vi "_LO_P_OPT2.vi"(5 "_LO_P_OPT":T3={"範囲配列"=[{"Start"=1.0, "Stop"=4.0, "Step"=0.05, "ｂｙ"="NEL VG"}, {"Start"=0.0, "Stop"=100.0, "Step"=4.0, "ｂｙ"="Motor"}, {"Start"=0.0, "Stop"=2.5, "Step"=0.1, "ｂｙ"="WCA VD"}], "Optimize"=0, "file_name"="LP_914.0_Tmin_100519.csv", "Save?"=FALSE, "measure"=1, "current(uA)"=60.0, "wait(ms)"=0, "IFfrq(GHz)"=8.0, "aveg"=10, "SISparam option"=2} {"SISparam option" items=["Volt and Current", "Volt only"]; "measure" items=["Pmax (only HOT)", "Tmin (HOT/COLD)", "C current"]; "Optimize" items=["Sweep", "黄金分割"]; "範囲配列"."Step" format="%.2f"; "範囲配列"."Stop" format="%.2f"; "範囲配列"."Start" format="%.2f"}, 6 "Control":T2={"GPIB_ATT"="28", "6501Dev#"=1, "GPIB_SP"="18", "GPIB_PM"="13", "GPIB_DSA"="11", "GPIB_DMM (TPD)"="23", "GPIB_MPI"="2", "mortor設定"=[{"Axis"=0, "ID"=0, "HIspeed"=200.0, "LOspeed"=100.0, "ACCEL(ms)"=100.0, "Sratio"=50.0, "フリーラン\n"=TRUE, "文字列"="DSB HOT/COLD"}, {"Axis"=1, "ID"=0, "HIspeed"=4.0, "LOspeed"=4.0, "ACCEL(ms)"=100.0, "Sratio"=50.0, "フリーラン\n"=TRUE, "文字列"="SubMM Att"}], "DATAパス"=path "Z:/band10/Labview_ALMA/MIX95/test", "DBパス "=path "Z:/band10/Labview_ALMA/MIX95/test", "comment"="P1_Tmin", "ColdCarts"="003601", "Th"=295.0, "Tc"=77.0, "Set_SIS_volt"=2.1, "Offset"=0.0, "control"=0, "FreqLO"=800.0, "Set_Mag_Cur"=800.0, "MPI offset(mm)"=22.99, "HOT/COLD"=0} {"HOT/COLD" items=["DSB", "SBR", "GainComp"]; "control" items=["CLOSE LOOP", "OPEN LOOP", "Not Control"]}, 7 "Bias_LO_equip":T1={"Node address"=19, "CAN Interface"="CAN0", "Cartridge band"=10, "Slave Node in"={"Address"=19, "Serial Number"=[16, 71, 55, 76, 1, 8, 0, -15]}, "ObjHandle out"=89653312, "POL"=0, "sb"=1, "GPIB_SM (SIS S,V)"="24", "GPIB_DMM (SIS I)"="22", "GPIB_SM (MAG I) "="25", "GPIB_SG(LO)"="19", "GPIB_PW (PAMP) "="6", "GPIB_TMP1(8ch)"="12", "GPIB_TMP2(2ch)  "="13", "WCA_avg"=10, "Rsen"=10.0, "BiasModule"=1, "LOModule "=1, "WCA_LO_FREQ_SET"={"YTO Low freq. [GHz]"=14.42, "YTO High freq. [GHz]"=17.7, "Kvco"=1, "Lock Pol."=0, "SET LO FREQ"=100.0, "Multiplier"=6.0, "YTO (HEX)"=2805, "YTO coarse( FREQ)"=16.666666, "NULL PLL INTEGRATOR"=TRUE}, "Res for"=0} {"Res for" items=["none", "series res", "parallel res"]; "WCA_LO_FREQ_SET"."YTO coarse( FREQ)" min=25 max=150 step=0.0001 format="%.3f"; "WCA_LO_FREQ_SET"."Multiplier" min=3 max=6 step=3; "WCA_LO_FREQ_SET"."SET LO FREQ" min=25 max=150 step=0.0001 format="%.3f"; "WCA_LO_FREQ_SET"."Lock Pol." items=["Lower", "Upper"]; "WCA_LO_FREQ_SET"."Kvco" items=["7.5MHz/V", "15MHz/V"]; "WCA_LO_FREQ_SET"."YTO High freq. [GHz]" format="%.3f"; "WCA_LO_FREQ_SET"."YTO Low freq. [GHz]" format="%.3f"; "LOModule" items=["Manual", "B10Lab LO", "WCA LO"]; "BiasModule" items=["B10Lab Bias", "WCA BiasModule"]; "Slave Node in"."Serial Number" format="%.0x"; "Slave Node in"."Address" format="%.0x"; "Cartridge band" max=10 step=1; "Node address" format="%.0x"}) -> (3 "結果":string="Tmin:1.200000,0.165295,-13.146817,-14.992015,334.790506")   [LabVIEW 2017]
uses:
  __sub_vi/WCA_NAOJ_sub_vi/WCA_Global.vi
panel:
  in  "タブ制御器":enum32{"ページ 1", "ページ 2"}(tab)=enum."ページ 2"
  out "minFx":dbl
  out "Fx":dbl
  out "I-Fx,Pc,Trx":cluster{dbl[], dbl[]}[](graph)=[{[153.7109375, 152.8717041015625, 153.0426025390625, 152.0904541015625, 152.197265625, 151.9866943359375, 151.7333984375, 151.7486572265625, 151.8402099609375, 150.8392333984375, 150.1068115234375, 149.4537353515625, 149.20654296875, 148.6541748046875, 148.1048583984375, 147.0977783203125, 146.6278076171875, 145.062255859375, 144.1864013671875, 143.5546875, 142.291259765625, 140.435791015625, 139.3341064453125, 137.652587890625, 135.430908203125, 133.2977294921875, 131.2896728515625, 129.229736328125, 125.5859375, 122.8668212890625, 118.975830078125, 114.666748046875, 110.8306884765625, 105.0506591796875, 100.1861572265625, 94.15283203125, 88.57421875, 81.0516357421875, 74.462890625, 66.8121337890625, 58.21533203125, 50.9368896484375, 43.5333251953125, 35.0921630859375, 28.1494140625, 21.0784912109375, 16.8365478515625, 13.39111328125, 10.7818603515625, 9.75341796875, 8.4869384765625, 8.978271484375, 8.062744140625, 7.7392578125, 8.43505859375, 7.8125, 7.6416015625, 7.7911376953125, 7.4615478515625, 8.099365234375, 7.89794921875], [247.32973404062736, 244.71794894153766, 242.21978128892934, 244.26842176336262, 241.49817645467988, 244.69487843477683, 242.06455494053583, 240.909445631355, 242.79140491659956, 239.77028849664566, 241.64156684519503, 239.88306106329682, 237.99335929764584, 239.24144610629918, 236.10546909689103, 231.85120086491656, 233.37184450401236, 233.2188877479738, 227.20848640844875, 225.76191805290316, 224.66247085466176, 223.0476471884519, 217.34620955182348, 215.60624700567845, 213.36678724449226, 210.01567868925287, 205.3448700334079, 204.4787981832116, 197.65786587642887, 194.28724400486016, 190.3621373523391, 185.96437875144585, 178.89458547136363, 178.034248343829, 167.74747224652654, 165.5095915634044, 161.1009828285456, 160.72538624241002, 155.93203338638352, 155.50825118261417, 154.03398781536052, 156.39456182240366, 163.7351172921269, 173.95257326151167, 197.43539223873222, 233.31332449649227, 302.2246629701954, 422.0785764312742, 621.6392407626414, 960.4947947838928, 1388.5150609483871, 2060.6013217578993, 2652.2540265629227, 3593.013865996171, 4493.467285194053, 5219.874679791377, 5585.654505061477, 7119.009590999049, 8443.334685028694, 7506.888534465469, 11478.336528646887]}, {[153.7109375, 152.8717041015625, 153.0426025390625, 152.0904541015625, 152.197265625, 151.9866943359375, 151.7333984375, 151.7486572265625, 151.8402099609375, 150.8392333984375, 150.1068115234375, 149.4537353515625, 149.20654296875, 148.6541748046875, 148.1048583984375, 147.0977783203125, 146.6278076171875, 145.062255859375, 144.1864013671875, 143.5546875, 142.291259765625, 140.435791015625, 139.3341064453125, 137.652587890625, 135.430908203125, 133.2977294921875, 131.2896728515625, 129.229736328125, 125.5859375, 122.8668212890625, 118.975830078125, 114.666748046875, 110.8306884765625, 105.0506591796875, 100.1861572265625, 94.15283203125, 88.57421875, 81.0516357421875, 74.462890625, 66.8121337890625, 58.21533203125, 50.9368896484375, 43.5333251953125, 35.0921630859375, 28.1494140625, 21.0784912109375, 16.8365478515625, 13.39111328125, 10.7818603515625, 9.75341796875, 8.4869384765625, 8.978271484375, 8.062744140625, 7.7392578125, 8.43505859375, 7.8125, 7.6416015625, 7.7911376953125, 7.4615478515625, 8.099365234375, 7.89794921875], [-14.7646696, -14.7654326, -14.7765426, -14.7599957, -14.7587965, -14.7416571, -14.7490545, -14.7393598, -14.7286239, -14.7227317, -14.7104064, -14.7025198, -14.6874695, -14.6799035, -14.6761139, -14.6736071, -14.6591382, -14.6331242, -14.6237809, -14.6066206, -14.5690542, -14.5442752, -14.5291663, -14.508835, -14.4645891, -14.4304201, -14.3839625, -14.3296729, -14.3047591, -14.2758504, -14.2368317, -14.1673127, -14.1313886, -14.0570048, -14.0333737, -13.9726864, -13.9307766, -13.8943843, -13.9278091, -13.9695187, -14.0952793, -14.286396, -14.5693598, -14.9860507, -15.5360188, -16.2362229, -17.0032381, -17.7253118, -18.2916002, -18.6658912, -18.9074033, -19.0515672, -19.1514628, -19.2030341, -19.2343409, -19.256989, -19.2916912, -19.2884725, -19.3062143, -19.3276449, -19.3006641]}, {[153.7109375, 152.8717041015625, 153.0426025390625, 152.0904541015625, 152.197265625, 151.9866943359375, 151.7333984375, 151.7486572265625, 151.8402099609375, 150.8392333984375, 150.1068115234375, 149.4537353515625, 149.20654296875, 148.6541748046875, 148.1048583984375, 147.0977783203125, 146.6278076171875, 145.062255859375, 144.1864013671875, 143.5546875, 142.291259765625, 140.435791015625, 139.3341064453125, 137.652587890625, 135.430908203125, 133.2977294921875, 131.2896728515625, 129.229736328125, 125.5859375, 122.8668212890625, 118.975830078125, 114.666748046875, 110.8306884765625, 105.0506591796875, 100.1861572265625, 94.15283203125, 88.57421875, 81.0516357421875, 74.462890625, 66.8121337890625, 58.21533203125, 50.9368896484375, 43.5333251953125, 35.0921630859375, 28.1494140625, 21.0784912109375, 16.8365478515625, 13.39111328125, 10.7818603515625, 9.75341796875, 8.4869384765625, 8.978271484375, 8.062744140625, 7.7392578125, 8.43505859375, 7.8125, 7.6416015625, 7.7911376953125, 7.4615478515625, 8.099365234375, 7.89794921875], [247.32973404062736, 244.71794894153766, 242.21978128892934, 244.26842176336262, 241.49817645467988, 244.69487843477683, 242.06455494053583, 240.909445631355, 242.79140491659956, 239.77028849664566, 241.64156684519503, 239.88306106329682, 237.99335929764584, 239.24144610629918, 236.10546909689103, 231.85120086491656, 233.37184450401236, 233.2188877479738, 227.20848640844875, 225.76191805290316, 224.66247085466176, 223.0476471884519, 217.34620955182348, 215.60624700567845, 213.36678724449226, 210.01567868925287, 205.3448700334079, 204.4787981832116, 197.65786587642887, 194.28724400486016, 190.3621373523391, 185.96437875144585, 178.89458547136363, 178.034248343829, 167.74747224652654, 165.5095915634044, 161.1009828285456, 160.72538624241002, 155.93203338638352, 155.50825118261417, 154.03398781536052, 156.39456182240366, 163.7351172921269, 173.95257326151167, 197.43539223873222, 233.31332449649227, 302.2246629701954, 422.0785764312742, 621.6392407626414, 960.4947947838928, 1388.5150609483871, 2060.6013217578993, 2652.2540265629227, 3593.013865996171, 4493.467285194053, 5219.874679791377, 5585.654505061477, 7119.009590999049, 8443.334685028694, 7506.888534465469, 11478.336528646887]}]
  out "X-I,Fx":cluster{dbl[], dbl[]}[](graph)=[{[1.0, 1.05, 1.1, 1.15, 1.2, 1.25, 1.3, 1.35, 1.4, 1.45, 1.5, 1.55, 1.6, 1.65, 1.7000000000000002, 1.75, 1.8, 1.85, 1.9, 1.9500000000000002, 2.0, 2.05, 2.1, 2.1500000000000004, 2.2, 2.25, 2.3, 2.35, 2.4000000000000004, 2.45, 2.5, 2.55, 2.6, 2.6500000000000004, 2.7, 2.75, 2.8, 2.85, 2.9000000000000004, 2.95, 3.0, 3.0500000000000003, 3.1, 3.15, 3.2, 3.25, 3.3000000000000003, 3.35, 3.4000000000000004, 3.45, 3.5, 3.5500000000000003, 3.6, 3.6500000000000004, 3.7, 3.75, 3.8000000000000003, 3.85, 3.9000000000000004, 3.95, 4.0], [153.7109375, 152.8717041015625, 153.0426025390625, 152.0904541015625, 152.197265625, 151.9866943359375, 151.7333984375, 151.7486572265625, 151.8402099609375, 150.8392333984375, 150.1068115234375, 149.4537353515625, 149.20654296875, 148.6541748046875, 148.1048583984375, 147.0977783203125, 146.6278076171875, 145.062255859375, 144.1864013671875, 143.5546875, 142.291259765625, 140.435791015625, 139.3341064453125, 137.652587890625, 135.430908203125, 133.2977294921875, 131.2896728515625, 129.229736328125, 125.5859375, 122.8668212890625, 118.975830078125, 114.666748046875, 110.8306884765625, 105.0506591796875, 100.1861572265625, 94.15283203125, 88.57421875, 81.0516357421875, 74.462890625, 66.8121337890625, 58.21533203125, 50.9368896484375, 43.5333251953125, 35.0921630859375, 28.1494140625, 21.0784912109375, 16.8365478515625, 13.39111328125, 10.7818603515625, 9.75341796875, 8.4869384765625, 8.978271484375, 8.062744140625, 7.7392578125, 8.43505859375, 7.8125, 7.6416015625, 7.7911376953125, 7.4615478515625, 8.099365234375, 7.89794921875]}, {[1.0, 1.05, 1.1, 1.15, 1.2, 1.25, 1.3, 1.35, 1.4, 1.45, 1.5, 1.55, 1.6, 1.65, 1.7000000000000002, 1.75, 1.8, 1.85, 1.9, 1.9500000000000002, 2.0, 2.05, 2.1, 2.1500000000000004, 2.2, 2.25, 2.3, 2.35, 2.4000000000000004, 2.45, 2.5, 2.55, 2.6, 2.6500000000000004, 2.7, 2.75, 2.8, 2.85, 2.9000000000000004, 2.95, 3.0, 3.0500000000000003, 3.1, 3.15, 3.2, 3.25, 3.3000000000000003, 3.35, 3.4000000000000004, 3.45, 3.5, 3.5500000000000003, 3.6, 3.6500000000000004, 3.7, 3.75, 3.8000000000000003, 3.85, 3.9000000000000004, 3.95, 4.0], [247.32973404062736, 244.71794894153766, 242.21978128892934, 244.26842176336262, 241.49817645467988, 244.69487843477683, 242.06455494053583, 240.909445631355, 242.79140491659956, 239.77028849664566, 241.64156684519503, 239.88306106329682, 237.99335929764584, 239.24144610629918, 236.10546909689103, 231.85120086491656, 233.37184450401236, 233.2188877479738, 227.20848640844875, 225.76191805290316, 224.66247085466176, 223.0476471884519, 217.34620955182348, 215.60624700567845, 213.36678724449226, 210.01567868925287, 205.3448700334079, 204.4787981832116, 197.65786587642887, 194.28724400486016, 190.3621373523391, 185.96437875144585, 178.89458547136363, 178.034248343829, 167.74747224652654, 165.5095915634044, 161.1009828285456, 160.72538624241002, 155.93203338638352, 155.50825118261417, 154.03398781536052, 156.39456182240366, 163.7351172921269, 173.95257326151167, 197.43539223873222, 233.31332449649227, 302.2246629701954, 422.0785764312742, 621.6392407626414, 960.4947947838928, 1388.5150609483871, 2060.6013217578993, 2652.2540265629227, 3593.013865996171, 4493.467285194053, 5219.874679791377, 5585.654505061477, 7119.009590999049, 8443.334685028694, 7506.888534465469, 11478.336528646887]}]
  out "Link済み":bool
  # "LO freq. [GHz]"
  # "YTO LOW\n/High Freq."
  # "ZERO Intgrtr"
  # "Node Address"
  # "Serial Number"
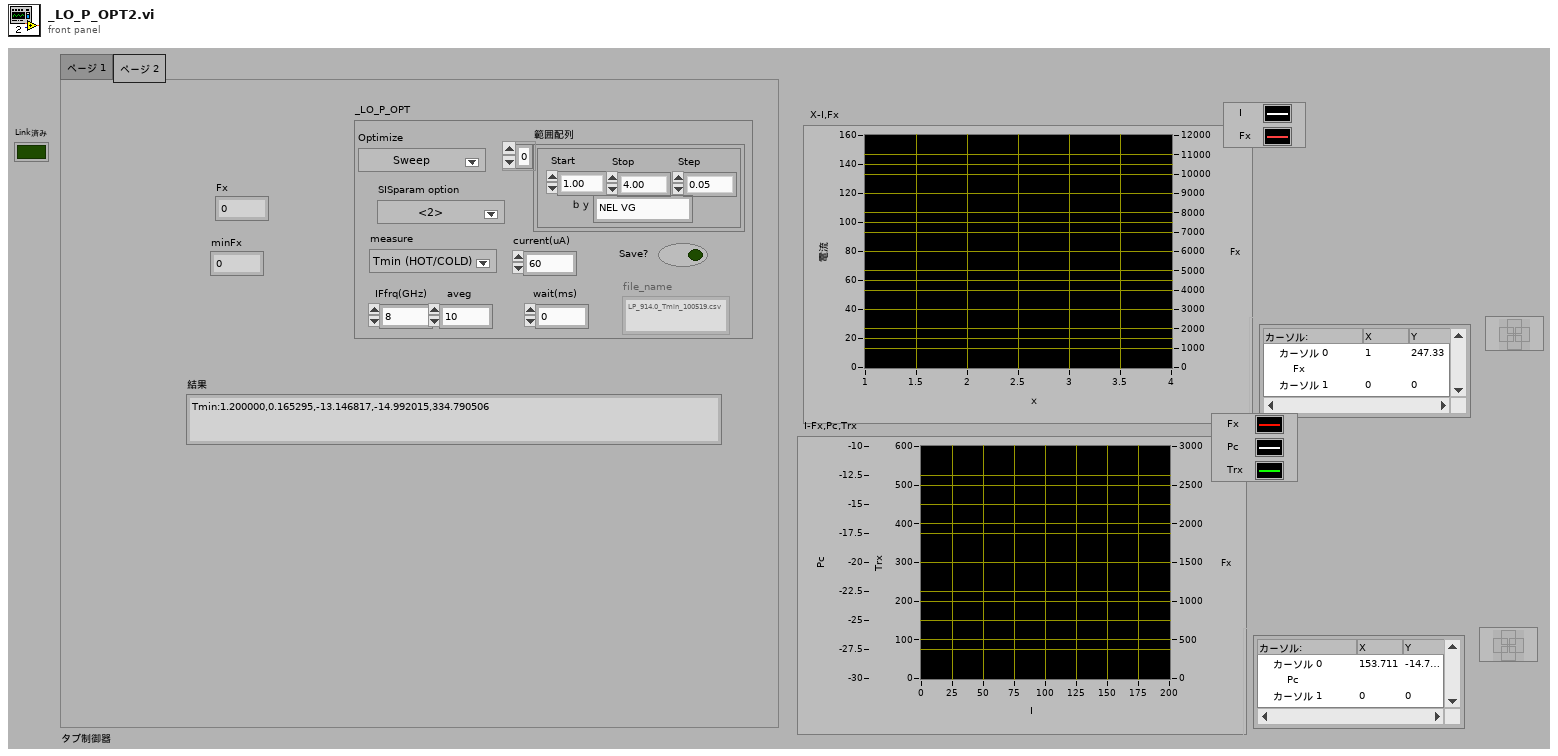
[diagram p1: front panel]
types:
  T1 = cluster{"Node address":u16, "CAN Interface":string, "Cartridge band":u32, "Slave Node in":cluster{"Address":i16, "Serial Number":i8[]}, "ObjHandle out":u32, "POL":u32, "sb":u32, "GPIB_SM (SIS S,V)":string, "GPIB_DMM (SIS I)":string, "GPIB_SM (MAG I) ":string, "GPIB_SG(LO)":string, "GPIB_PW (PAMP) ":string, "GPIB_TMP1(8ch)":string, "GPIB_TMP2(2ch)  ":string, "WCA_avg":i32, "Rsen":dbl, "BiasModule":u16, "LOModule ":u16, "WCA_LO_FREQ_SET":cluster{"YTO Low freq. [GHz]":sgl, "YTO High freq. [GHz]":sgl, "Kvco":u16, "Lock Pol.":u16, "SET LO FREQ":sgl, "Multiplier":sgl, "YTO (HEX)":u16, "YTO coarse( FREQ)":sgl, "NULL PLL INTEGRATOR":bool}, "Res for":u16}
  T2 = cluster{"GPIB_ATT":string, "6501Dev#":i16, "GPIB_SP":string, "GPIB_PM":string, "GPIB_DSA":string, "GPIB_DMM (TPD)":string, "GPIB_MPI":string, "mortor設定":cluster{"Axis":i16, "ID":i16, "HIspeed":dbl, "LOspeed":dbl, "ACCEL(ms)":dbl, "Sratio":dbl, "フリーラン\n":bool, "文字列":string}[], "DATAパス":path, "DBパス ":path, "comment":string, "ColdCarts":string, "Th":dbl, "Tc":dbl, "Set_SIS_volt":dbl, "Offset":dbl, "control":u16, "FreqLO":dbl, "Set_Mag_Cur":dbl, "MPI offset(mm)":dbl, "HOT/COLD":u16}
  T3 = cluster{"範囲配列":cluster{"Start":dbl, "Stop":dbl, "Step":dbl, "ｂｙ":string}[], "Optimize":u16, "file_name":string, "Save?":bool, "measure":u16, "current(uA)":dbl, "wait(ms)":i32, "IFfrq(GHz)":dbl, "aveg":i32, "SISparam option":u16}
  T4 = cluster{"Axis":i16, "ID":i16, "HIspeed":dbl, "LOspeed":dbl, "ACCEL(ms)":dbl, "Sratio":dbl, "フリーラン\n":bool, "文字列":string}[]
  T5 = cluster{"Axis":i16, "ID":i16, "HIspeed":dbl, "LOspeed":dbl, "ACCEL(ms)":dbl, "Sratio":dbl, "フリーラン\n":bool, "文字列":string}
  T6 = cluster{"Start":dbl, "Stop":dbl, "Step":dbl, "ｂｙ":string}[]
  T7 = cluster{"Start":dbl, "Stop":dbl, "Step":dbl, "ｂｙ":string}
  T8 = cluster{"PA_A_DRAIN_V":sgl, "PA_A_DRAIN_C":sgl, "PA_A_GATE_V":sgl, "PA_B_DRAIN_V":sgl, "PA_B_DRAIN_C":sgl, "PA_B_GATE_V":sgl, "PA_3V_SUPPLY_V":sgl, "PA_5V_MON":sgl}
  T9 = cluster{"出力配列[0]":dbl, "出力配列[1]":dbl, "出力配列[2]":dbl, "出力配列[3]":dbl, "出力配列[4]":dbl, "出力配列[5]":dbl, "出力配列[6]":dbl}
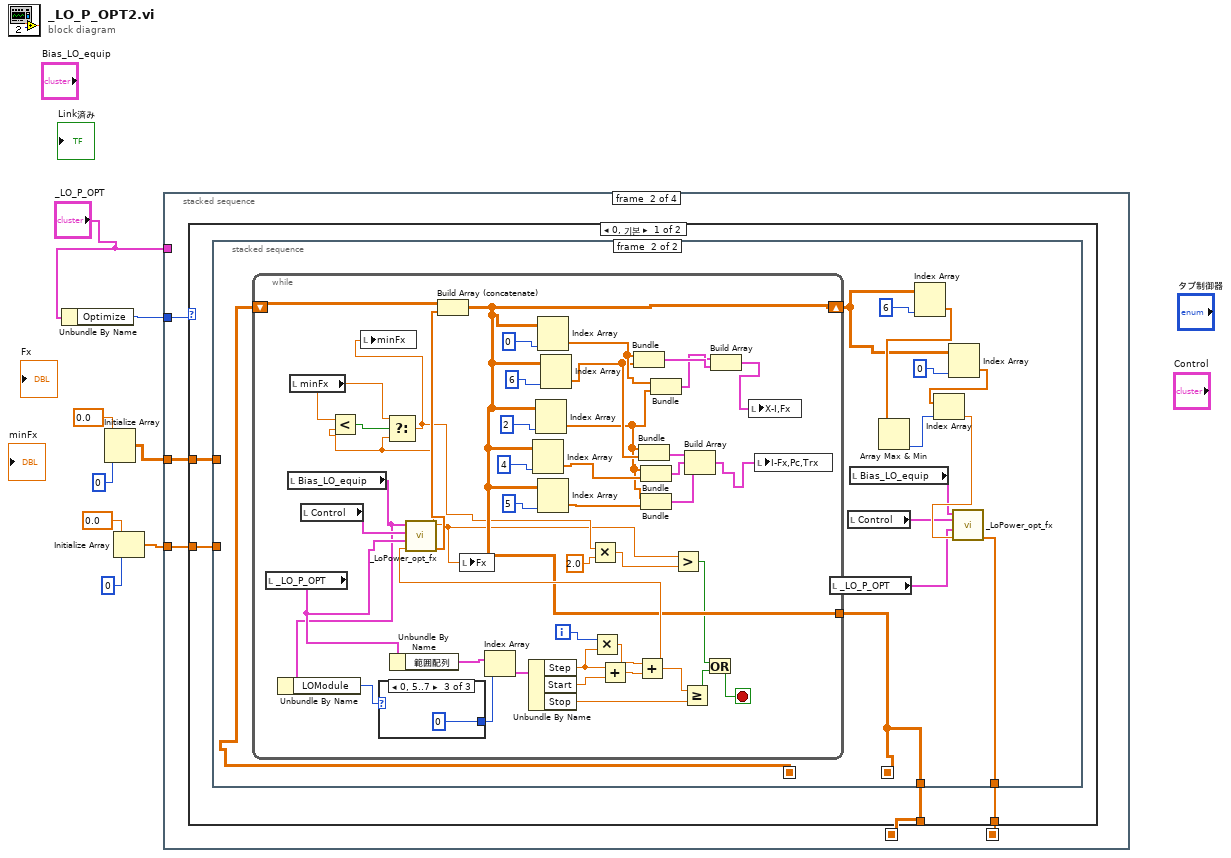
[diagram p0: block diagram]
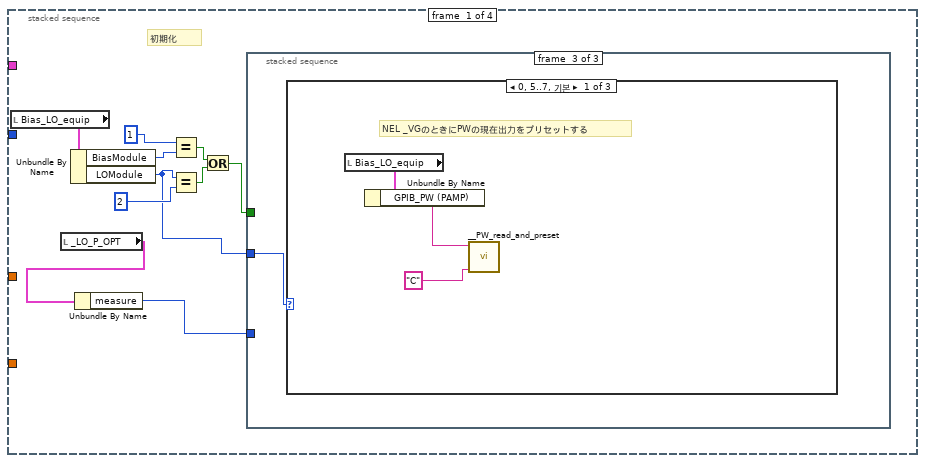
[diagram p2: hidden frame]
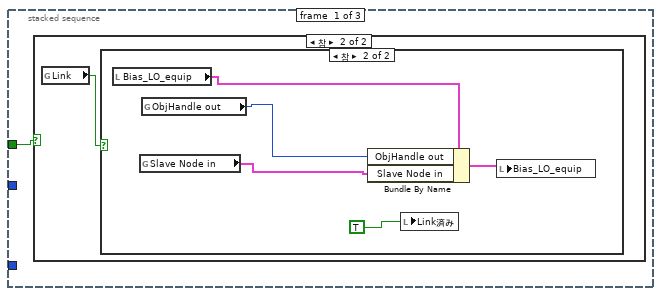
[diagram p3: hidden frame]
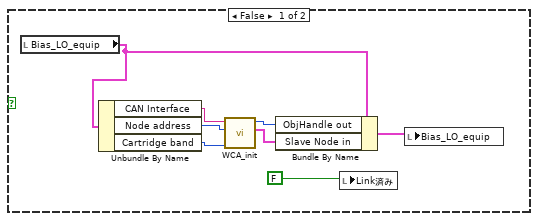
[diagram p5: hidden frame]
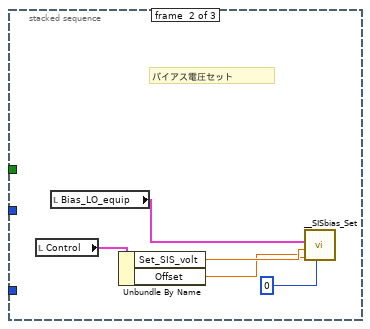
[diagram p6: hidden frame]
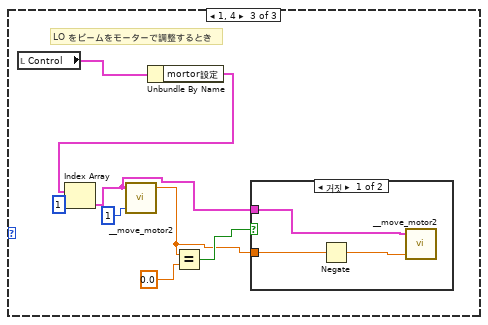
[diagram p8: hidden frame]
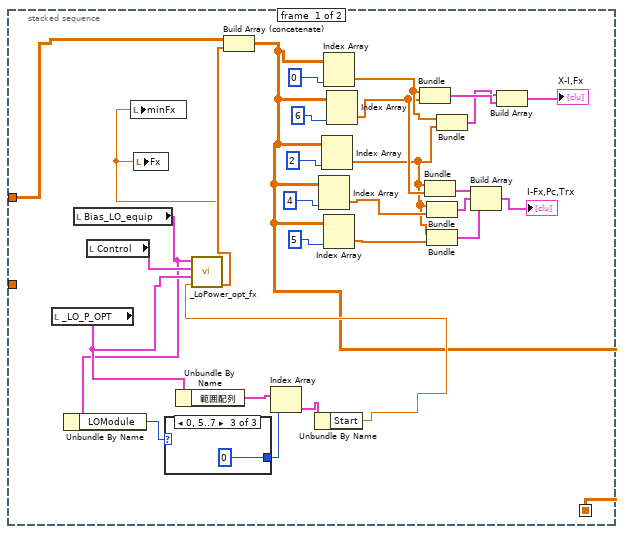
[diagram p10: hidden frame]
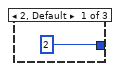
[diagram p11: hidden frame]
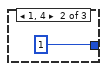
[diagram p12: hidden frame]
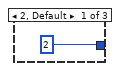
[diagram p13: hidden frame]
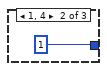
[diagram p14: hidden frame]
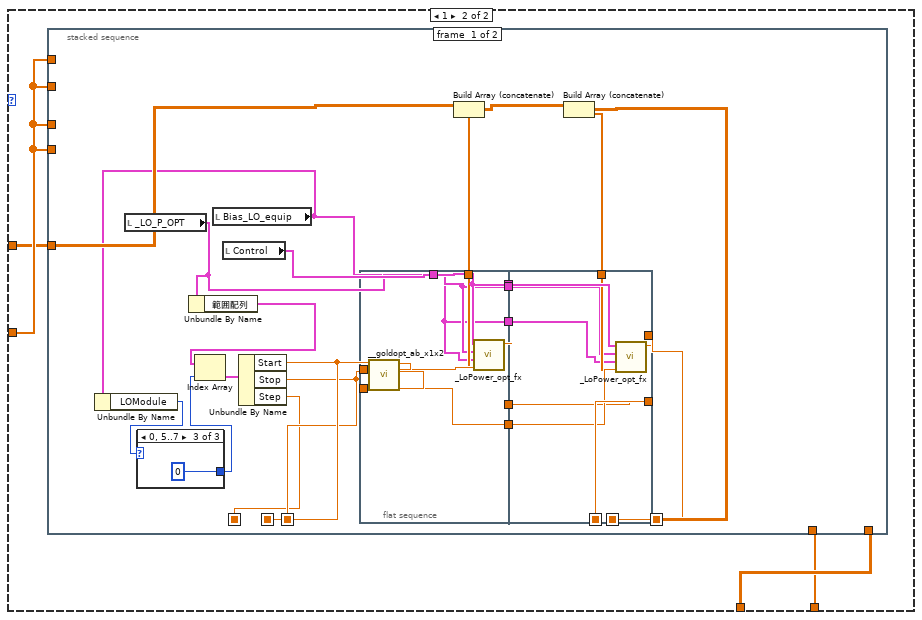
[diagram p15: hidden frame]
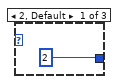
[diagram p16: hidden frame]
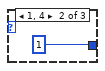
[diagram p17: hidden frame]
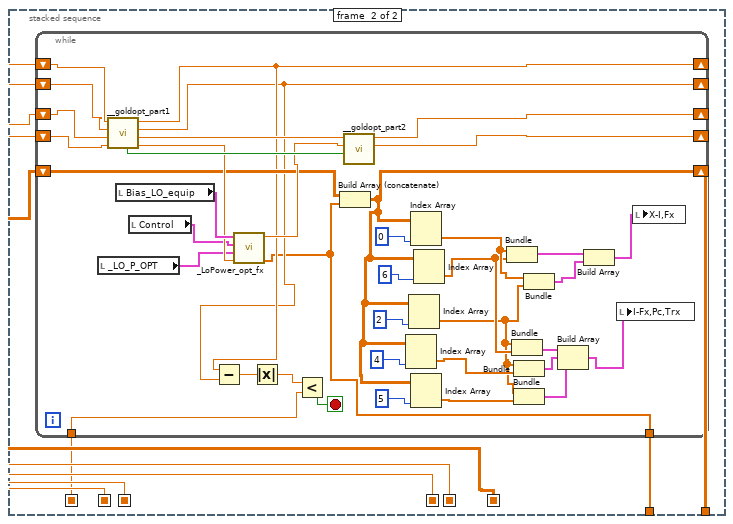
[diagram p18: hidden frame]
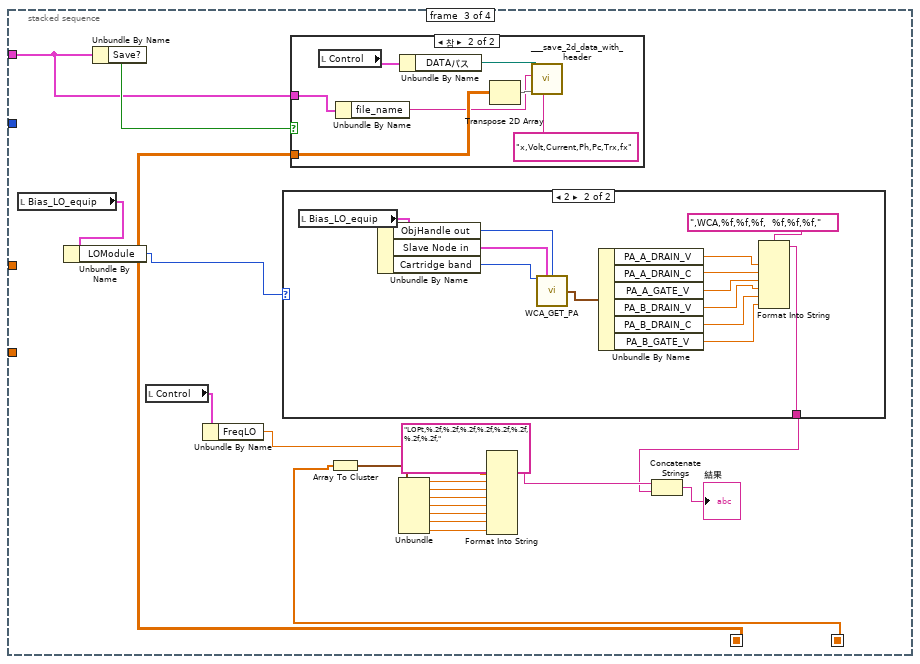
[diagram p19: hidden frame]
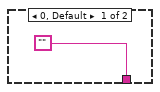
[diagram p20: hidden frame]
diagram:
  w2 = 0
  n1 = Unbundle By Name("_LO_P_OPT") -> ("Optimize"=w4:u16)
  n2 = Initialize Array(0.0, w2, w2) -> (w1:dbl[][])
  n3 = Initialize Array(0.0, 0) -> (w6:dbl[])
  n4 = stacked-sequence {
    seq-local: [_ w56 _ _] -> [_ _ w264 _]
    seq-local: [_ w54 _ _] -> [_ _ w262 _]
    tunnel: w6 -> [_ w57 _ _]
    tunnel: "_LO_P_OPT" -> [_ _ w263 _]
    tunnel: w4 -> [_ w58 _ _]
    tunnel: w1 -> [_ w55 _ _]
    frame #0 {
      # "初期化"
      n5 = local read "Bias_LO_equip"() -> (w13:T1)
      n6 = local read "_LO_P_OPT"() -> (w11:T3)
      n7 = Unbundle By Name(w13) -> ("BiasModule"=w14:u16, "LOModule"=w9:u16)
      n8 = Unbundle By Name(w11) -> ("measure"=w10:u16)
      n9 = Equal?(x=1, y=w14) -> (x = y?=w17:bool)
      n10 = Equal?(x=w9, y=2) -> (x = y?=w18:bool)
      n11 = Or(x=w17, y=w18) -> (x .or. y?=w12:bool)
      n12 = stacked-sequence {
        tunnel: w12 -> [w19 _ _]
        tunnel: w10 -> [_ _ _]
        tunnel: w9 -> [_ _ w39]
        frame #0 {
          n13 = case shown="참" w19 {
            frame False {
            }
            frame True {
              n14 = global read "WCA_Global.vi" "Link"() -> (w20:bool)
              n15 = case shown="참" w20 {
                frame False {
                  n16 = local read "Bias_LO_equip"() -> (w22:T1)
                  n17 = Unbundle By Name(w22) -> ("CAN Interface"=w26:string, "Node address"=w25:u16, "Cartridge band"=w24:u32)
                  n18 = call "WCA_init.vi"("Cartridge band"=w24, "Node address"=w25, "CAN Interface"=w26) -> ("Slave Node in"=w27:cluster{"Address":i16, "Serial Number":i8[]}, "ObjHandle out"=w28:u32)  [unwired: 4 in, 3 out]
                  n19 = Bundle By Name(cluster=w22, "ObjHandle out"=w28, "Slave Node in"=w27) -> (w23:T1)
                  n20 = local write "Link済み"(FALSE) -> ()
                  n21 = local write "Bias_LO_equip"(w23) -> ()
                }
                frame True {
                  n22 = local read "Bias_LO_equip"() -> (w32:T1)
                  n23 = global read "WCA_Global.vi" "Slave Node in"() -> (w30:cluster{"Address":i16, "Serial Number":i8[]})
                  n24 = global read "WCA_Global.vi" "ObjHandle out"() -> (w31:u32)
                  n25 = Bundle By Name(cluster=w32, "ObjHandle out"=w31, "Slave Node in"=w30) -> (w33:T1)
                  n26 = local write "Link済み"(TRUE) -> ()
                  n27 = local write "Bias_LO_equip"(w33) -> ()
                }
              }
            }
          }
        }
        frame #1 {
          # "バイアス電圧セット"
          n28 = local read "Control"() -> (w36:T2)
          n29 = local read "Bias_LO_equip"() -> (w38:T1)
          n30 = Unbundle By Name(w36) -> ("Set_SIS_volt"=w35:dbl, "Offset"=w34:dbl)
          n31 = call "__SISbias_Set.vi"("SIS　Mode"=0, "Offset"=w34, "Set_V"=w35, "Bias_LO_equip"=w38) -> ()  [unwired: 7 in, 1 out]
        }
        frame #2 {
          n32 = case shown="0, 5..7, 기본" w39 {
            frame 0, 5..7, Default {
              # "NEL _VGのときにPWの現在出力をプリセットする"
              n33 = local read "Bias_LO_equip"() -> (w42:T1)
              n34 = Unbundle By Name(w42) -> ("GPIB_PW (PAMP)"=w41:string)
              n35 = call "__PW_read_and_preset.vi"("MAXCh（A,B,C,D）"="C", "GPIB"=w41) -> ()  [unwired: 10 in]
            }
            frame 2 {
            }
            frame 1, 4 {
              # "LO をビームをモーターで調整するとき"
              n36 = local read "Control"() -> (w47:T2)
              n37 = Unbundle By Name(w47) -> ("mortor設定"=w48:T4)
              n38 = Index Array(array=w48, index=1) -> (element=w43:T5)
              n39 = call "__move_motor2.vi"("Moving distance"=1, "motor setup"=w43) -> ("counter"=w44:dbl)  [unwired: 2 in, 1 out]
              n40 = Equal?(x=w44, y=0.0) -> (x = y?=w50:bool)
              n41 = case shown="거짓" w50 {
                tunnel: w44 -> [w53 _]
                tunnel: w43 -> [w51 _]
                frame False {
                  n42 = Negate(x=w53) -> (-x=w52:dbl)
                  n43 = call "__move_motor2.vi"("Moving distance"=w52, "motor setup"=w51) -> ()  [unwired: 2 in, 2 out]
                }
                frame True {
                }
              }
            }
          }
        }
      }
    }
    frame #1 {
      n44 = case shown="0, 기본" w58 {
        tunnel: w57 -> [w62 w157]
        tunnel: [w61 w155] -> w56
        tunnel: w55 -> [w60 w156]
        tunnel: [w59 w154] -> w54
        frame 0, Default {
          n45 = stacked-sequence {
            seq-local: [_ w105] -> [_ _]
            seq-local: [w64 _] -> [_ w95]
            tunnel: w62 -> [_ _]
            tunnel: [_ w105] -> w61
            tunnel: w60 -> [w91 _]
            tunnel: [_ w97] -> w59
            frame #0 {
              n46 = local read "_LO_P_OPT"() -> (w69:T3)
              n47 = local read "Bias_LO_equip"() -> (w68:T1)
              n48 = Unbundle By Name(w68) -> ("LOModule"=w67:u16)
              n49 = local read "Control"() -> (w70:T2)
              n50 = case shown="0, 5..7" w67 {
                tunnel: [2 1 0] -> w66
                frame 2, Default {
                }
                frame 1, 4 {
                }
                frame 0, 5..7 {
                }
              }
              n51 = Unbundle By Name(w69) -> ("範囲配列"=w90:T6)
              n52 = Index Array(array=w90, index=w66) -> (element=w89:T7)
              n53 = Unbundle By Name(w89) -> ("Start"=w65:dbl)
              n54 = call "_LoPower_opt_fx.vi"("ｘ"=w65, "_LO_P_OPT"=w69, "Control"=w70, "Bias_LO_equip"=w68) -> ("出力配列"=w85:dbl[], "fx"=w63:dbl)  [unwired: 6 in]
              n55 = local write "minFx"(w63) -> ()
              n56 = local write "Fx"(w63) -> ()
              n57 = Build Array (concatenate)(w91, w85) -> (w64:dbl[][])
              n58 = Index Array(array=w64, index (col)=4) -> (element=w81:dbl[])  [unwired: 1 in]
              n59 = Index Array(array=w64, index (col)=2) -> (element=w80:dbl[])  [unwired: 1 in]
              n60 = Index Array(array=w64, index (col)=0) -> (element=w84:dbl[])  [unwired: 1 in]
              n61 = Index Array(array=w64, index (col)=5) -> (element=w79:dbl[])  [unwired: 1 in]
              n62 = Index Array(array=w64, index (col)=6) -> (element=w82:dbl[])  [unwired: 1 in]
              n63 = Bundle(w84, w82) -> (w72:cluster{dbl[], dbl[]})  [unwired: 1 in]
              n64 = Bundle(w80, w82) -> (w88:cluster{dbl[], dbl[]})  [unwired: 1 in]
              n65 = Bundle(w80, w81) -> (w87:cluster{dbl[], dbl[]})  [unwired: 1 in]
              n66 = Bundle(w80, w79) -> (w86:cluster{dbl[], dbl[]})  [unwired: 1 in]
              n67 = Bundle(w84, w80) -> (w71:cluster{dbl[], dbl[]})  [unwired: 1 in]
              n68 = Build Array(w88, w87, w86) -> (→"I-Fx,Pc,Trx":cluster{dbl[], dbl[]}[])
              n69 = Build Array(w71, w72) -> (→"X-I,Fx":cluster{dbl[], dbl[]}[])
            }
            frame #1 {
              n70 = while {
                tunnel: [w138] -> w105
                shift-right: [w138] -> w99
                shift-left: w95 -> [w140]
                i -> [w147]
                stop <- w115 stop-if-true
                n71 = local read "_LO_P_OPT"() -> (w124:T3)
                n72 = local read "Bias_LO_equip"() -> (w123:T1)
                n73 = Unbundle By Name(w123) -> ("LOModule"=w122:u16)
                n74 = local read "minFx"() -> (w117:dbl)
                n75 = local read "Control"() -> (w125:T2)
                n76 = case shown="0, 5..7" w122 {
                  tunnel: [2 1 0] -> w121
                  frame 2, Default {
                  }
                  frame 1, 4 {
                  }
                  frame 0, 5..7 {
                  }
                }
                n77 = Unbundle By Name(w124) -> ("範囲配列"=w150:T6)
                n78 = Index Array(array=w150, index=w121) -> (element=w149:T7)
                n79 = Unbundle By Name(w149) -> ("Step"=w119:dbl, "Start"=w148:dbl, "Stop"=w145:dbl)
                n80 = Multiply(x=w147, y=w119) -> (x*y=w146:dbl)
                n81 = Add(x=w119, y=w148) -> (x+y=w120:dbl)
                n82 = Add(x=w146, y=w120) -> (x+y=w144:dbl)
                n83 = call "_LoPower_opt_fx.vi"("ｘ"=w144, "_LO_P_OPT"=w124, "Control"=w125, "Bias_LO_equip"=w123) -> ("出力配列"=w139:dbl[], "fx"=w111:dbl)  [unwired: 6 in]
                n84 = Less?(x=w117, y=w111) -> (x < y?=w118:bool)
                n85 = Select(t=w117, s=w118, f=w111) -> (s? t:f=w112:dbl)
                n86 = local write "minFx"(w112) -> ()
                n87 = Build Array (concatenate)(w140, w139) -> (w138:dbl[][])
                n88 = local write "Fx"(w111) -> ()
                n89 = Index Array(array=w138, index (col)=4) -> (element=w135:dbl[])  [unwired: 1 in]
                n90 = Index Array(array=w138, index (col)=2) -> (element=w134:dbl[])  [unwired: 1 in]
                n91 = Index Array(array=w138, index (col)=0) -> (element=w137:dbl[])  [unwired: 1 in]
                n92 = Index Array(array=w138, index (col)=5) -> (element=w133:dbl[])  [unwired: 1 in]
                n93 = Index Array(array=w138, index (col)=6) -> (element=w136:dbl[])  [unwired: 1 in]
                n94 = Multiply(x=w112, y=2.0) -> (x*y=w110:dbl)
                n95 = Bundle(w137, w136) -> (w127:cluster{dbl[], dbl[]})  [unwired: 1 in]
                n96 = Bundle(w134, w136) -> (w143:cluster{dbl[], dbl[]})  [unwired: 1 in]
                n97 = Bundle(w134, w135) -> (w142:cluster{dbl[], dbl[]})  [unwired: 1 in]
                n98 = Bundle(w134, w133) -> (w141:cluster{dbl[], dbl[]})  [unwired: 1 in]
                n99 = Bundle(w137, w134) -> (w126:cluster{dbl[], dbl[]})  [unwired: 1 in]
                n100 = Greater?(x=w111, y=w110) -> (0:w113:bool)
                n101 = Greater Or Equal?(x=w144, y=w145) -> (x >= y?=w114:bool)
                n102 = Build Array(w143, w142, w141) -> (w108:cluster{dbl[], dbl[]}[])
                n103 = Or(x=w113, y=w114) -> (x .or. y?=w115:bool)
                n104 = Build Array(w126, w127) -> (w109:cluster{dbl[], dbl[]}[])
                n105 = local write "X-I,Fx"(w109) -> ()
                n106 = local write "I-Fx,Pc,Trx"(w108) -> ()
              }
              n107 = local read "_LO_P_OPT"() -> (w96:T3)
              n108 = local read "Control"() -> (w100:T2)
              n109 = local read "Bias_LO_equip"() -> (w106:T1)
              n110 = Index Array(array=w99, index (col)=6) -> (element=w104:dbl[])  [unwired: 1 in]
              n111 = Array Max & Min(array=w104) -> (min index (indices)=w98:i32)  [unwired: 3 out]
              n112 = Index Array(array=w99, index (col)=0) -> (element=w103:dbl[])  [unwired: 1 in]
              n113 = Index Array(array=w103, index=w98) -> (element=w107:dbl)
              n114 = call "_LoPower_opt_fx.vi"("ｘ"=w107, "_LO_P_OPT"=w96, "Control"=w100, "Bias_LO_equip"=w106) -> ("出力配列"=w97:dbl[])  [unwired: 6 in, 1 out]
            }
          }
        }
        frame 1 {
          n115 = stacked-sequence {
            seq-local: [w169 _] -> [_ w206]
            seq-local: [w168 _] -> [_ w205]
            seq-local: [w171 _] -> [_ w202]
            seq-local: [w166 _] -> [_ w204]
            seq-local: [w165 _] -> [_ w203]
            seq-local: [w164 _] -> [_ w201]
            tunnel: w157 -> [_ _]
            tunnel: w157 -> [_ _]
            tunnel: w157 -> [_ _]
            tunnel: w157 -> [_ _]
            tunnel: w156 -> [w176 _]
            tunnel: [_ w200] -> w155
            tunnel: [_ w199] -> w154
            frame #0 {
              n116 = local read "_LO_P_OPT"() -> (w162:T3)
              n117 = Unbundle By Name(w162) -> ("範囲配列"=w181:T6)
              n118 = local read "Bias_LO_equip"() -> (w158:T1)
              n119 = Unbundle By Name(w158) -> ("LOModule"=w159:u16)
              n120 = case shown="0, 5..7" w159 {
                tunnel: [2 1 0] -> w160
                frame 2, Default {
                }
                frame 1, 4 {
                }
                frame 0, 5..7 {
                }
              }
              n121 = Index Array(array=w181, index=w160) -> (element=w180:T7)
              n122 = local read "Control"() -> (w179:T2)
              n123 = Unbundle By Name(w180) -> ("Start"=w169:dbl, "Stop"=w168:dbl, "Step"=w164:dbl)
              n124 = flat-sequence {
                tunnel: w162 -> [w185]
                tunnel: w179 -> [w186]
                tunnel: w158 -> [w190]
                tunnel: w172 -> [w191]
                tunnel: [w190] -> w178
                tunnel: w170 -> [w189]
                tunnel: [w189] -> w177
                tunnel: [w188] -> w175
                tunnel: [w187] -> w167
                tunnel: [w186] -> w163
                tunnel: [w185] -> w161
                tunnel: w178 -> [w198]
                tunnel: w177 -> [w197]
                tunnel: [w196] -> w173
                tunnel: w167 -> [w195]
                tunnel: [w195] -> w166
                tunnel: [w194] -> w165
                tunnel: w163 -> [w193]
                tunnel: w161 -> [w192]
                frame #0 {
                  n125 = call "_LoPower_opt_fx.vi"("ｘ"=w191, "_LO_P_OPT"=w185, "Control"=w186, "Bias_LO_equip"=w190) -> ("出力配列"=w188:dbl[], "fx"=w187:dbl)  [unwired: 6 in]
                }
                frame #1 {
                  n126 = call "_LoPower_opt_fx.vi"("ｘ"=w197, "_LO_P_OPT"=w192, "Control"=w193, "Bias_LO_equip"=w198) -> ("出力配列"=w196:dbl[], "fx"=w194:dbl)  [unwired: 6 in]
                }
              }
              n127 = call "__goldopt_ab_x1x2.vi"("bi"=w168, "ai"=w169) -> ("x2"=w170:dbl, "x1"=w172:dbl)  [unwired: 8 in]
              n128 = Build Array (concatenate)(w176, w175) -> (w174:dbl[][])
              n129 = Build Array (concatenate)(w174, w173) -> (w171:dbl[][])
            }
            frame #1 {
              n130 = while {
                shift-right: [w214] -> _
                shift-left: w206 -> [w245]
                shift-right: [w213] -> _
                shift-left: w205 -> [w244]
                shift-right: [w236] -> _
                shift-left: w204 -> [w243]
                shift-right: [w235] -> _
                shift-left: w203 -> [w242]
                shift-right: [w219] -> w200
                shift-left: w202 -> [w220]
                tunnel: w201 -> [w212]
                tunnel: [w209] -> w199
                stop <- w211 stop-if-true
                n131 = local read "_LO_P_OPT"() -> (w207:T3)
                n132 = call "__goldopt_part1.vi"("f2"=w242, "f1"=w243, "bi"=w244, "ai"=w245) -> ("x"=w238:dbl, "fout"=w241:dbl, "bi 2"=w213:dbl, "ai 2"=w214:dbl, "f2>f1"=w240:bool)  [unwired: 3 in]
                n133 = local read "Bias_LO_equip"() -> (w239:T1)
                n134 = local read "Control"() -> (w210:T2)
                n135 = Subtract(x=w214, y=w213) -> (x-y=w215:dbl)
                n136 = call "_LoPower_opt_fx.vi"("ｘ"=w238, "_LO_P_OPT"=w207, "Control"=w210, "Bias_LO_equip"=w239) -> ("出力配列"=w209:dbl[], "fx"=w237:dbl)  [unwired: 6 in]
                n137 = Absolute Value(x=w215) -> (abs(x)=w216:dbl)
                n138 = Less?(x=w216, y=w212) -> (x < y?=w211:bool)
                n139 = Build Array (concatenate)(w220, w209) -> (w219:dbl[][])
                n140 = call "__goldopt_part2.vi"("f2>f1"=w240, "f_changed"=w237, "f_notchange"=w241) -> ("f2"=w235:dbl, "f1"=w236:dbl)  [unwired: 7 in]
                n141 = Index Array(array=w219, index (col)=4) -> (element=w227:dbl[])  [unwired: 1 in]
                n142 = Index Array(array=w219, index (col)=2) -> (element=w226:dbl[])  [unwired: 1 in]
                n143 = Index Array(array=w219, index (col)=0) -> (element=w229:dbl[])  [unwired: 1 in]
                n144 = Index Array(array=w219, index (col)=5) -> (element=w225:dbl[])  [unwired: 1 in]
                n145 = Index Array(array=w219, index (col)=6) -> (element=w228:dbl[])  [unwired: 1 in]
                n146 = Bundle(w229, w228) -> (w234:cluster{dbl[], dbl[]})  [unwired: 1 in]
                n147 = Bundle(w226, w228) -> (w232:cluster{dbl[], dbl[]})  [unwired: 1 in]
                n148 = Bundle(w226, w227) -> (w231:cluster{dbl[], dbl[]})  [unwired: 1 in]
                n149 = Bundle(w226, w225) -> (w230:cluster{dbl[], dbl[]})  [unwired: 1 in]
                n150 = Bundle(w229, w226) -> (w233:cluster{dbl[], dbl[]})  [unwired: 1 in]
                n151 = Build Array(w232, w231, w230) -> (w217:cluster{dbl[], dbl[]}[])
                n152 = Build Array(w234, w233) -> (w218:cluster{dbl[], dbl[]}[])
                n153 = local write "I-Fx,Pc,Trx"(w217) -> ()
                n154 = local write "X-I,Fx"(w218) -> ()
              }
            }
          }
        }
      }
    }
    frame #2 {
      n155 = local read "Bias_LO_equip"() -> (w247:T1)
      n156 = Unbundle By Name(w247) -> ("LOModule"=w246:u16)
      n157 = Unbundle By Name(w263) -> ("Save?"=w265:bool)
      n158 = local read "Control"() -> (w256:T2)
      n159 = Unbundle By Name(w256) -> ("FreqLO"=w255:dbl)
      n160 = case shown="2" w246 {
        tunnel: ["" w267] -> w257
        frame 0, Default {
        }
        frame 2 {
          n161 = local read "Bias_LO_equip"() -> (w279:T1)
          n162 = Unbundle By Name(w279) -> ("ObjHandle out"=w277:u32, "Slave Node in"=w278:cluster{"Address":i16, "Serial Number":i8[]}, "Cartridge band"=w276:u32)
          n163 = call "WCA_GET_PA.vi"("Cartridge Band"=w276, "Slave Node in"=w278, "ObjHandle in"=w277) -> ("GET_PA"=w275:T8)  [unwired: 10 in, 2 out]
          n164 = Unbundle By Name(w275) -> ("PA_A_DRAIN_V"=w273:sgl, "PA_A_DRAIN_C"=w272:sgl, "PA_A_GATE_V"=w271:sgl, "PA_B_DRAIN_V"=w270:sgl, "PA_B_DRAIN_C"=w269:sgl, "PA_B_GATE_V"=w268:sgl)
          n165 = Format Into String(format string=",WCA,%f,%f,%f,  %f,%f,%f,", w273, w272, w271, w270, w269, w268) -> (resulting string=w267:string)  [unwired: 2 in, 1 out]
        }
      }
      n166 = case shown="참" w265 {
        tunnel: w264 -> [_ w286]
        tunnel: w263 -> [_ w284]
        frame False {
        }
        frame True {
          n167 = local read "Control"() -> (w281:T2)
          n168 = Unbundle By Name(w284) -> ("file_name"=w283:string)
          n169 = Unbundle By Name(w281) -> ("DATAパス"=w280:path)
          n170 = Transpose 2D Array(2D array=w286) -> (transposed array=w285:dbl[][])
          n171 = call "___save_2d_data_with_header.vi"("ヘッダー"="x,Volt,Current,Ph,Pc,Trx,fx", "配列"=w285, "file_name"=w283, "パス"=w280) -> ()  [unwired: 7 in, 1 out]
        }
      }
      n172 = Array To Cluster(array=w262) -> (cluster=w261:T9)
      n173 = Unbundle(w261) -> ("出力配列[0]"=w254:dbl, "出力配列[1]"=w253:dbl, "出力配列[2]"=w252:dbl, "出力配列[3]"=w251:dbl, "出力配列[4]"=w250:dbl, "出力配列[5]"=w249:dbl, "出力配列[6]"=w248:dbl)
      n174 = Format Into String(format string="LOPt,%.2f,%.2f,%.2f,%.2f,%.2f,%.2f,%.2f,%.2f,", w255, w254, w253, w252, w251, w250, w249, w248) -> (resulting string=w258:string)  [unwired: 2 in, 1 out]
      n175 = Concatenate Strings(w258, w257) -> (→"結果":string)
    }
    frame #3 {
      n176 = local read "Bias_LO_equip"() -> (w287:T1)
      n177 = Unbundle By Name(w287) -> ("BiasModule"=w288:u16, "LOModule"=w290:u16)
      n178 = Equal?(x=1, y=w288) -> (x = y?=w292:bool)
      n179 = Equal?(x=w290, y=2) -> (x = y?=w293:bool)
      n180 = Or(x=w292, y=w293) -> (x .or. y?=w294:bool)
      n181 = case shown="참" w294 {
        frame False {
        }
        frame True {
          n182 = local read "Link済み"() -> (w295:bool)
          n183 = case shown="거짓" w295 {
            frame False {
              n184 = local read "Bias_LO_equip"() -> (w297:T1)
              n185 = local write "Link済み"(FALSE) -> ()
              n186 = Unbundle By Name(w297) -> ("ObjHandle out"=w296:u32)
              n187 = call "WCA_CAN_close.vi"("ObjHandle in"=w296) -> ()  [unwired: 14 in, 1 out]
            }
            frame True {
            }
          }
        }
      }
    }
  }
